vi "gap_table_to_uncompressed_waveform.vi"(0 "Variable Names":string[](array[string]), 1 "Clock Rate":dbl, 3 "Timing Sequence Control (ms)":string[][](array[string]), 5 "Current Value Array":dbl[](array[numeric]), 11 "HSDIO Settings.Hardware alignment quantum\n(in samples)":u16=1, 14 "units/sec (ms=1000)":dbl) -> (4 "Transitions":u32[](array[numeric]), 6 "Data":u32[](array[numeric]) format="%04b", 8 "Waveform was padded":bool, 10 "output waveform":digitaldata, 15 "Waveform Duration (ms)":dbl)   [LabVIEW 2013]
uses:
  <vilib>/gmath/NI_Gmath.lvlib
panel:
  out "Gap Timing Sequence [ms]":dbl[][](array[numeric])
  out "Absolute Timing Sequence [samples]":dbl[][](array[numeric])
  out "Flattened Transition Array":u64[](array[numeric])
  out "Redunancy Removed":u64[](array[numeric])
  out "Non-Redundant Sorted Array":u64[](array[numeric])
  out "Last Element Reduced":u32[](array[numeric])
  out "# of Channels":i32
  out "# transitions per channel":i32
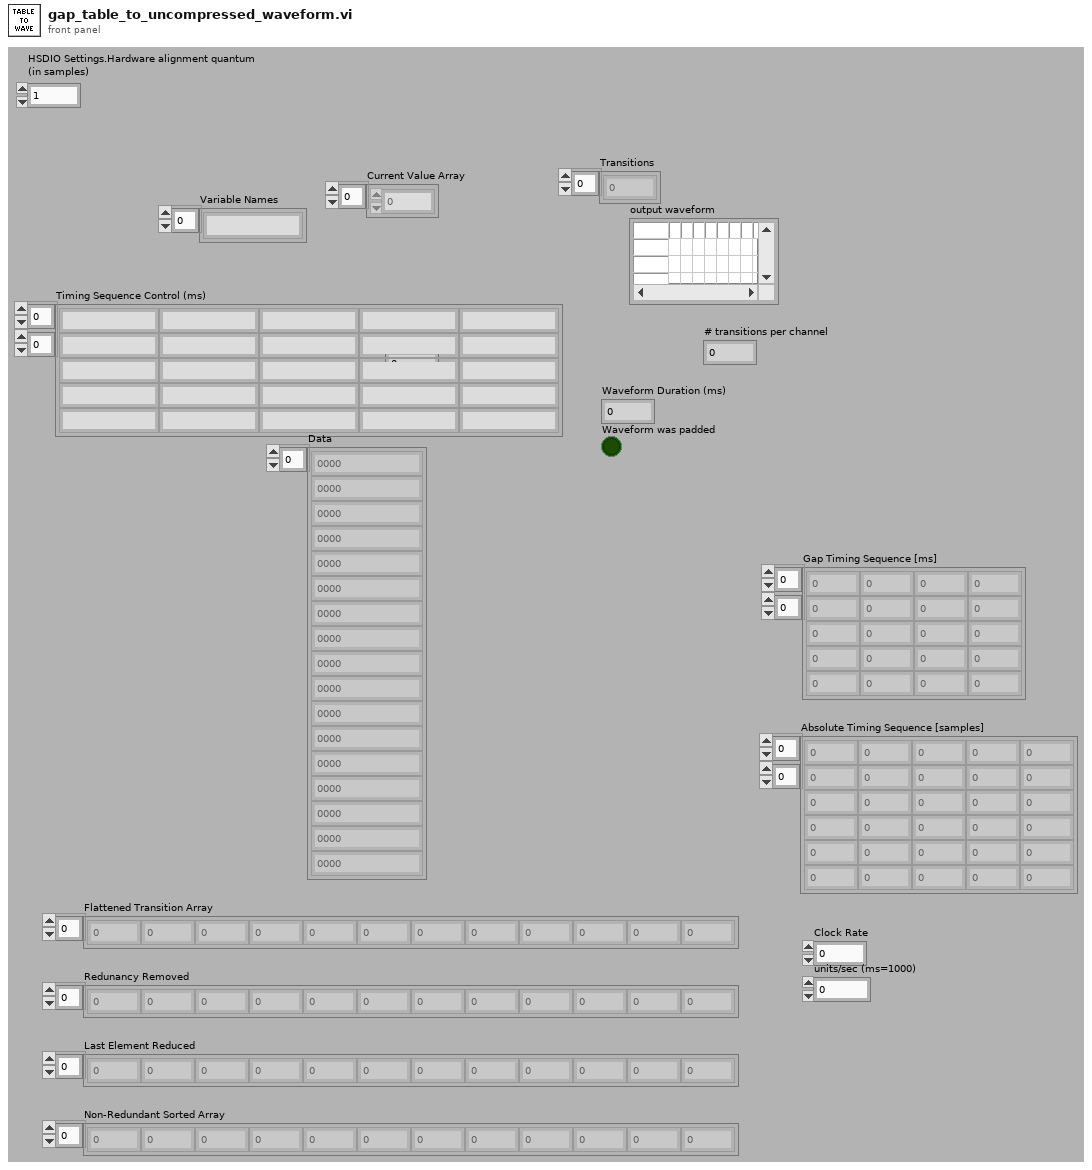
[diagram p1: front panel]
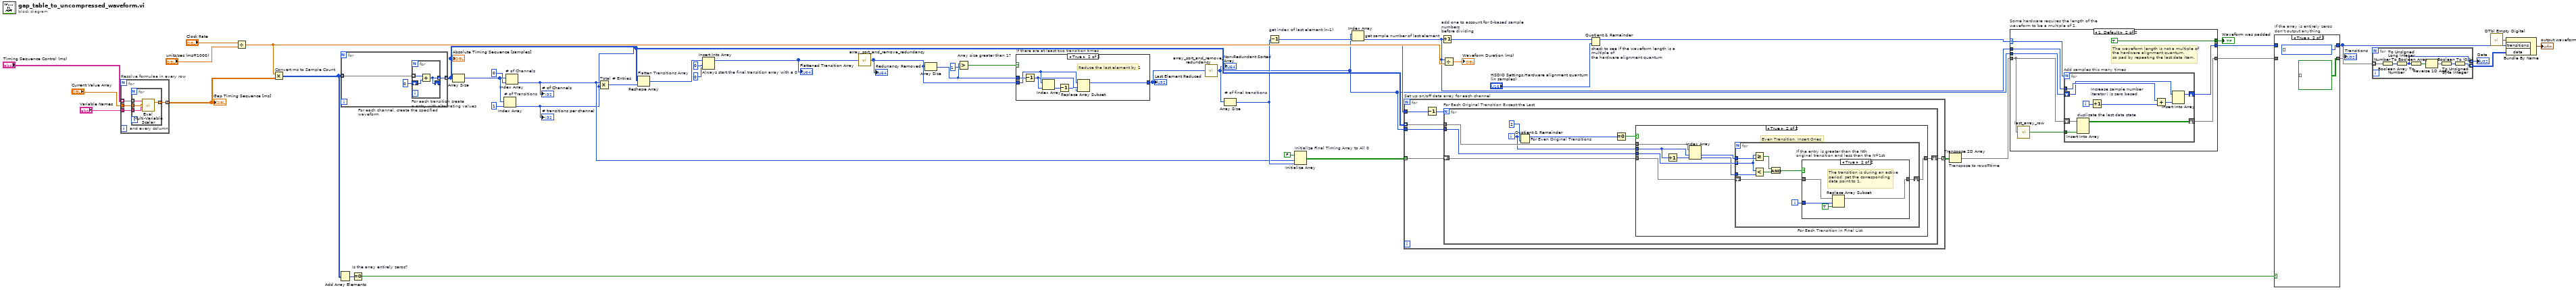
[diagram p0: block diagram]
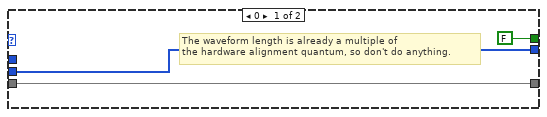
[diagram p3: hidden frame]
diagram:
  n1 = for "Resolve formulae in every row" {
    tunnel: "Timing Sequence Control (ms)" -> [w51] mode=indexing
    tunnel: [w48] -> w9 mode=indexing
    tunnel: "Variable Names" -> [w50]
    tunnel: "Current Value Array" -> [w49]
    n2 = for "and every column" {
      tunnel: w51 -> [w55] mode=indexing
      tunnel: [w53] -> w48 mode=indexing
      tunnel: w50 -> [w54]
      tunnel: w49 -> [w52]
      n3 = call <vilib>:"Eval Multi-Variable Scalar.vi"("Variables"=w54, "X Values"=w52, "formula"=w55) -> ("y value"=w53:dbl)  [unwired: 1 in, 1 out]
    }
  }
  "Gap Timing Sequence [ms]" <- w9
  n4 = Divide(x="Clock Rate", y="units/sec (ms=1000)") -> (x/y=w29:dbl)
  n5 = Multiply "Convert ms to Sample Count"(x=w29, y=w9) -> (x*y=w7:u32[][])
  n6 = Add Array Elements(numeric array=w7) -> (sum=w8:u32)
  n7 = for "For each channel, create the specified waveform" {
    tunnel: w7 -> [w58] mode=indexing
    tunnel: [w56] -> w35 mode=indexing
    n8 = for "For each transition create \na entry with alternating values" {
      tunnel: w58 -> [w61] mode=indexing
      shift-right: [w59] -> _
      shift-left: u64 0 -> [w60]
      tunnel: [w59] -> w56 mode=indexing
      n9 = Add(x=w61, y=w60) -> (x+y=w59:u64)
    }
  }
  "Absolute Timing Sequence [samples]" <- w35
  n10 = Equal To 0? "Is the array entirely zeros?"(x=w8) -> (x = 0?=w6:bool)
  n11 = Array Size(array=w35) -> (size(s)=w47:i32[])
  n12 = Index Array "# of Transitions"(array=w47, index=1) -> (element=w15:i32)
  "# transitions per channel" <- w15
  n13 = Index Array "# of Channels"(array=w47, index=0) -> (element=w16:i32)
  "# of Channels" <- w16
  n14 = Multiply "Total # Entries"(x=w16, y=w15) -> (x*y=w44:i32)
  n15 = Reshape Array "Flatten Transitions Array"(w35, w44) -> (w42:u64[])
  n16 = Insert Into Array "Always start the final transition array with a 0"(array=w42, index=u32 0, new element=u64 0 ("new element/subarray")) -> (w39:u64[])
  "Flattened Transition Array" <- w39
  n17 = call "array_sort_and_remove_redundancy.vi"("Full Array"=w39) -> ("Non-Redundant Sorted Array"=w27:u32[])
  "Redunancy Removed" <- w27
  n18 = Array Size(array=w27) -> (size(s)=w26:i32)
  n19 = Greater? "Array size greater than 1?"(x=w26, y=1) -> (0:w25:bool)
  n20 = case "If there are at least two transition times" shown="True" w25 {
    tunnel: w27 -> [w62 w67]
    tunnel: w26 -> [_ w68]
    tunnel: [w62 w63] -> w38
    frame False {
      # "The only element is zero, just leave it."
    }
    frame True {
      # "Reduce the last element by 1"
      n21 = Decrement(x=w68) -> (x-1=w66:i32)
      n22 = Index Array(array=w67, index=w66) -> (element=w65:u32)
      n23 = Decrement(x=w65) -> (x-1=w64:u32)
      n24 = Replace Array Subset "Replace Array Subset"(array=w67, new element=w64, index=w66) -> (w63:u32[])
    }
  }
  "Last Element Reduced" <- w38
  n25 = call "array_sort_and_remove_redundancy.vi"("Full Array"=w38) -> ("Non-Redundant Sorted Array"=w10:u32[])
  "Non-Redundant Sorted Array" <- w10
  n26 = Array Size "# of final transitions"(array=w10) -> (size(s)=w22:i32)
  n27 = Decrement "get index of last element (n-1)"(x=w22) -> (x-1=w30:i32)
  n28 = Initialize Array "Initialize Final Timing Array to All 0"(FALSE, w16, w22) -> (w36:bool[][])
  n29 = Index Array "get sample number of last element"(array=w10, index=w30) -> (element=w13:u32)
  n30 = for "Set up on/off data array for each channel" {
    tunnel: w36 -> [w74] mode=indexing
    tunnel: w35 -> [w73] mode=indexing
    tunnel: [w72] -> w21 mode=indexing
    tunnel: w10 -> [w71]
    tunnel: w15 -> [w69]
    n31 = Decrement(x=w69) -> (x-1=w70:i32)
    n32 = for "For Each Original Transition Except the Last" {
      N: w70 -> [_]
      tunnel: w73 -> [w80]
      tunnel: w71 -> [w75]
      shift-right: [w79] -> w72
      shift-left: w74 -> [w81]
      i -> [w76]
      n33 = Quotient & Remainder "For Even Original Transitions"(x=w76, y=2) -> (x-y*floor(x/y)=w78:i32)  [unwired: 1 out]
      n34 = Equal To 0?(x=w78) -> (x = 0?=w77:bool)
      n35 = case shown="True" w77 {
        tunnel: w81 -> [w83 w91]
        tunnel: w80 -> [_ w88]
        tunnel: [w83 w90] -> w79
        tunnel: w76 -> [_ w89]
        tunnel: w75 -> [_ w86]
        frame False {
          # "Odd Transition, Do Nothing"
        }
        frame True {
          # "Even Transition, Insert Ones"
          n36 = Increment(x=w89) -> (x+1=w85:i32)
          n37 = Index Array "Index Array"(array=w88, index #1=w89, index #2=w85) -> (element #1=w87:u64, element #2=w84:u64)
          n38 = for "For Each Transition in Final List" {
            tunnel: w84 -> [w99]
            tunnel: w87 -> [w98]
            tunnel: w86 -> [w97] mode=indexing
            shift-right: [w100] -> w90
            shift-left: w91 -> [w93]
            i -> [w92]
            n39 = Greater Or Equal?(x=w97, y=w98) -> (x >= y?=w96:bool)
            n40 = Less?(x=w97, y=w99) -> (x < y?=w95:bool)
            n41 = And(x=w96, y=w95) -> (x .and. y?=w94:bool)
            n42 = case "If the entry is greater than the Nth\noriginal transition and less than the N+1st" shown="True" w94 {
              tunnel: w93 -> [w101 w105]
              tunnel: [w101 w104] -> w100
              tunnel: w92 -> [_ w103]
              frame False {
                # "Do nothing."
              }
              frame True {
                # "The transition is during an active period, set the corresponding data point to 1."
                n43 = Replace Array Subset(array=w105, new element=TRUE, index=w103) -> (w104:bool[])
              }
            }
          }
        }
      }
    }
  }
  n44 = Increment "add one to account for 0-based sample numbers\nbefore dividing"(x=w13) -> (x+1=w12:u32)
  n45 = Divide(x=w13, y=w29) -> (x/y=→"Waveform Duration (ms)":dbl)
  n46 = Quotient & Remainder "check to see if the waveform length is a multiple of\nthe hardware alignment quantum"(x=w12, y="HSDIO Settings.Hardware alignment quantum\n(in samples)") -> (x-y*floor(x/y)=w11:u32)  [unwired: 1 out]
  n47 = Transpose 2D Array "Transpose to rows=time"(2D array=w21) -> (transposed array=w19:bool[][])
  n48 = case "Some hardware requires the length of the\nwaveform to be a multiple of 2." shown="1, Default" w11 {
    selector: w11 -> [_ w115]
    tunnel: w13 -> [_ w114]
    tunnel: w10 -> [w108 w113]
    tunnel: [w108 w112] -> w5
    tunnel: w19 -> [w107 w111]
    tunnel: [w107 w109] -> w2
    tunnel: [FALSE TRUE] -> w24
    frame 0 {
      # "The waveform length is already a multiple of\nthe hardware alignment quantum, so don't do anything."
    }
    frame 1, Default {
      # "The waveform length is not a multiple of\nthe hardware alignment quantum,\nso pad by repeating the last data item."
      n49 = call "last_array_row.vi"("array"=w111) -> ("subarray"=w110:bool[])
      n50 = for "Add samples this many times" {
        N: w115 -> [_]
        tunnel: w114 -> [w124]
        shift-right: [w120] -> w112
        shift-left: w113 -> [w121]
        tunnel: w110 -> [w118]
        shift-right: [w117] -> w109
        shift-left: w111 -> [w119]
        i -> [w125]
        n51 = Insert Into Array "duplicate the last data state"(array=w119, new element=w118) -> (w117:bool[][])  [unwired: 2 in]
        n52 = Increment "Increase sample number\niterator i is zero based"(x=w125) -> (x+1=w123:i32)
        n53 = Add(x=w124, y=w123) -> (x+y=w122:u32)
        n54 = Insert Into Array(array=w121, new element=w122) -> (w120:u32[])  [unwired: 1 in]
      }
    }
  }
  "Waveform was padded" <- w24
  n55 = case "If the array is entirely zeros\ndon't output anything" shown="True" w6 {
    tunnel: w5 -> [w127 _]
    tunnel: [w127 u32[] [] ("Non-Redundant Sorted Array")] -> w4
    tunnel: w2 -> [w126 _]
    tunnel: [w126 bool[][] []] -> w1
    frame False {
    }
    frame True {
    }
  }
  "Transitions" <- w4
  n56 = for {
    tunnel: w1 -> [w136] mode=indexing
    tunnel: [w134] -> w20 mode=indexing
    tunnel: [w130] -> w3 mode=indexing
    n57 = Boolean Array To Number(Boolean array=w136) -> (number=w135:u32)
    n58 = To Unsigned Long Integer(number=w135) -> (unsigned 32bit integer=w134:u32)
    n59 = Number To Boolean Array(number=w134) -> (Boolean array=w133:bool[])
    n60 = Reverse 1D Array(array=w133) -> (reversed array=w132:bool[])
    n61 = Boolean To (0,1)(Boolean=w132) -> (0, 1=w131:i16[])
    n62 = To Unsigned Byte Integer(number=w131) -> (unsigned 8bit integer=w130:u8[])
  }
  "Data" <- w20
  n63 = call <vilib>:"DTbl Empty Digital.vi"() -> ("digital data"=w18:digitaldata)  [unwired: 5 in]
  n64 = Bundle By Name(cluster=w18, "transitions"=w4, "data"=w3) -> (→"output waveform":digitaldata)
